vi "Practica_3.vi"() -> ()   [LabVIEW 2018]
uses:
  <vilib>/Instr/_visa.llb/VISA Configure Serial Port (Instr).vi
panel:
  out "Waveform Chart":dbl(graph)
  out "*(type *) &x 3":u16
  out "*(type *) &x 2":u16
  out "*(type *) &x":u16
  in  "stop":bool
  in  "baud rate (9600)":u32=9600
  in  "VISA resource name":refnum<visa-resource-name>
  out "read buffer":string
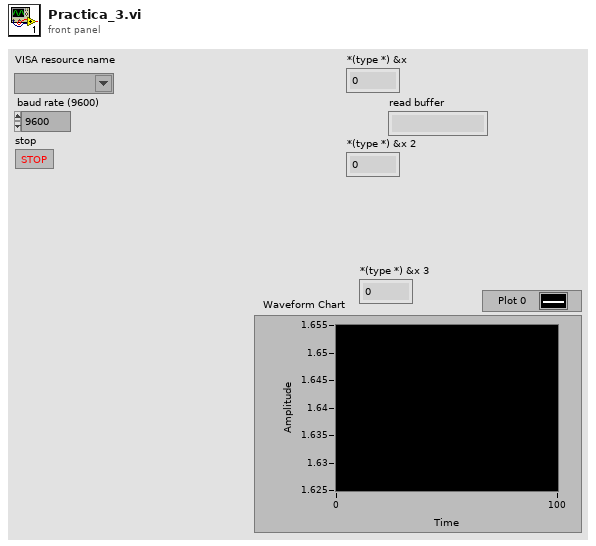
[diagram p1: front panel]
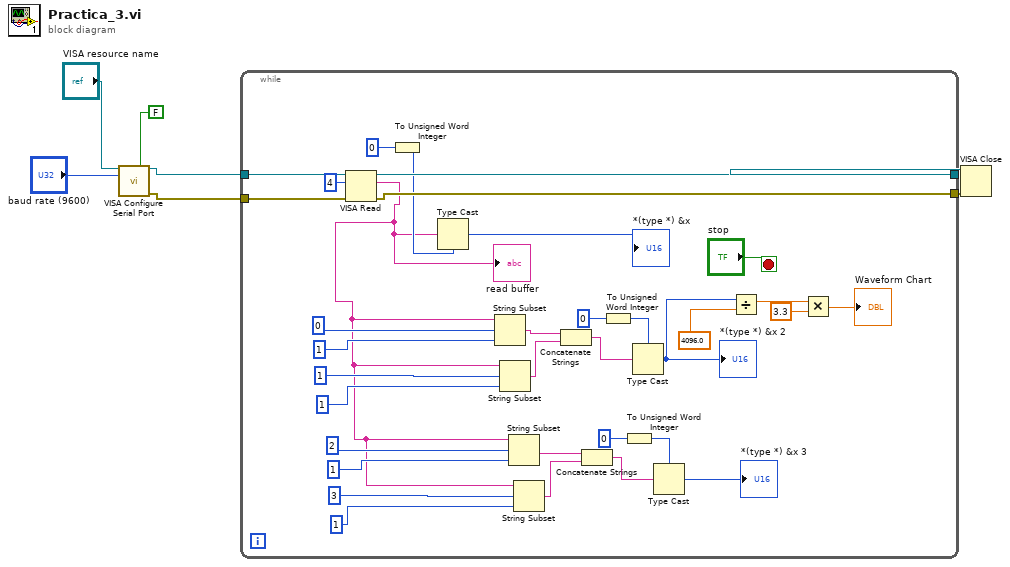
[diagram p0: block diagram]
diagram:
  n1 = call-poly "VISA Configure Serial Port"("VISA resource name"="VISA resource name", "Enable Termination\nChar (T)"=FALSE ("Enable Termination\nChar (T)"), "baud rate (9600)"="baud rate (9600)") -> ("VISA resource name out"=w7:refnum<visa-resource-name>, "error out"=w6:errorcluster)  [unwired: 11 in]
  n2 = while {
    tunnel: w7 -> [w41]
    tunnel: [w40] -> w5
    tunnel: w6 -> [w39]
    tunnel: [w38] -> w4
    stop <- "stop" stop-if-true
    n3 = VISA Read(VISA resource name=w41, byte count=u32 4, error in (no error)=w39) -> (VISA resource name out=w40:refnum<visa-resource-name>, read buffer=w22:string, error out=w38:errorcluster)  [unwired: 1 out]
    "read buffer" <- w22
    n4 = To Unsigned Word Integer(number=u8 0) -> (unsigned 16bit integer=w36:u16)
    n5 = Type Cast(type=w36, x=w22) -> (*(type *) &x=→"*(type *) &x":u16)
    n6 = String Subset(string=w22, offset (0)=0, length (rest)=1 ("length (rest)")) -> (substring=w20:string)
    n7 = String Subset(string=w22, offset (0)=1, length (rest)=1 ("length (rest)")) -> (substring=w19:string)
    n8 = String Subset(string=w22, offset (0)=2, length (rest)=1 ("length (rest)")) -> (substring=w14:string)
    n9 = String Subset(string=w22, offset (0)=3, length (rest)=1 ("length (rest)")) -> (substring=w13:string)
    n10 = Concatenate Strings(w20, w19) -> (w28:string)
    n11 = Concatenate Strings(w14, w13) -> (w16:string)
    n12 = To Unsigned Word Integer(number=u8 0) -> (unsigned 16bit integer=w29:u16)
    n13 = To Unsigned Word Integer(number=u8 0) -> (unsigned 16bit integer=w15:u16)
    n14 = Type Cast(type=w29, x=w28) -> (*(type *) &x=w11:u16)
    "*(type *) &x 2" <- w11
    n15 = Type Cast(type=w15, x=w16) -> (*(type *) &x=→"*(type *) &x 3":u16)
    n16 = Divide(x=w11, y=4096.0) -> (x/y=w10:dbl)
    n17 = Multiply(x=w10, y=3.3) -> (x*y=→"Waveform Chart":dbl)
  }
  n18 = VISA Close(VISA resource name=w5, error in (no error)=w4) -> ()  [unwired: 1 out]
